vi "ApplicaFunzCorr_INPUT.vi"(0 "Array":T1[](array[typedef])) -> (7 "Array Cluster Corretto":T1[](array[typedef]))   [LabVIEW 2016]
uses:
  <vilib>/Analysis/6fits.llb/Curve Fitting Criteria.ctl
  <vilib>/Utility/file.llb/Read Delimited Spreadsheet (string).vi
  <vilib>/Analysis/polynomials.llb/Scalar Polynomial Evaluation (DBL).vi
  <vilib>/Analysis/polynomials.llb/Polynomial Plot (Range).vi
  <vilib>/Analysis/NI_AALPro.lvlib
panel:
  in  "Cluster Misura / Unità":T1
  out "Misure da correggere":dbl[](array[numeric])
  out "Misure Corrette":dbl[](array[numeric])
  out "Graph":cluster{"Ramp Pattern":dbl[], "P(A)":dbl[]}[](graph)
  out "Y":dbl[](array[numeric])
  out "X":dbl[](array[numeric])
  out "Subarray dati selezionati":string[][](array[string])
  out "Lettura file di testo":string[][](array[string])
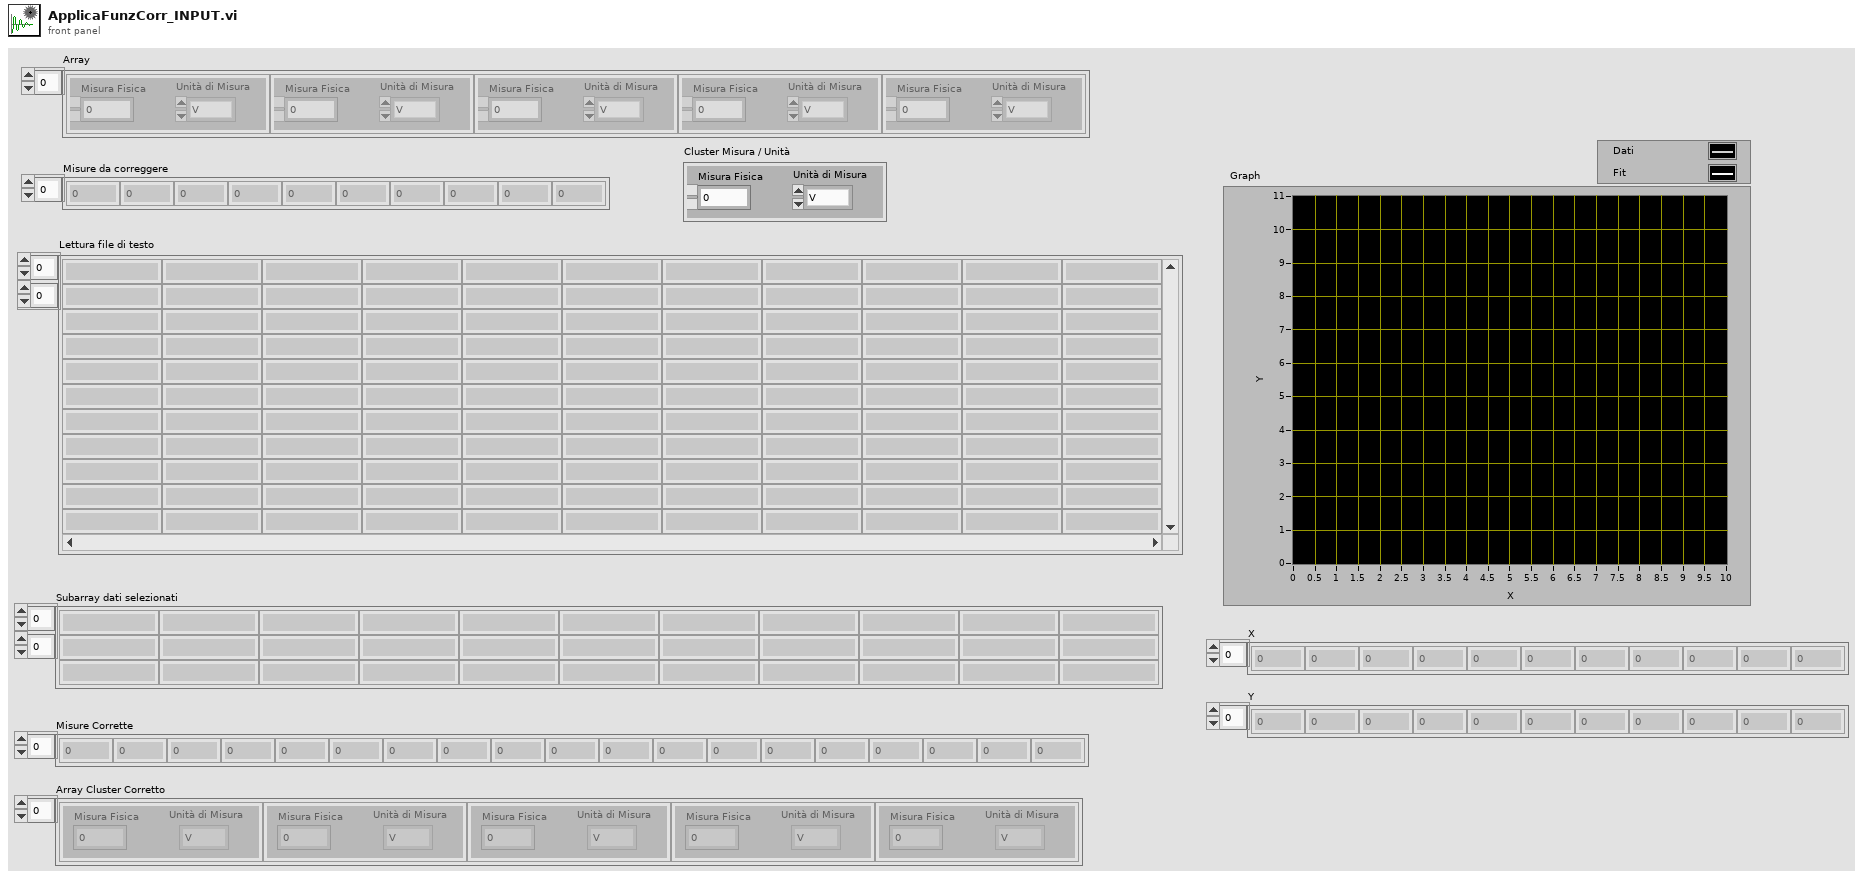
[diagram p1: front panel]
types:
  T1 = typedef "ClusterMisura_e_Unità_INPUT.ctl" = cluster{"Misura Fisica":dbl, "Unità di Misura":T2}
  T2 = typedef "UnitàMisura.ctl" = enum16{"V", "mA", "Bar", "RPM", "m3/s", "m3/min", "m3/h", "l/s", "l/min", "in3/min", "ft3/min", "gpm", "igpm", "igph"}
  T3 = typedef "NI_AALPro.lvlib/Curve Fitting Criteria.ctl" = u16
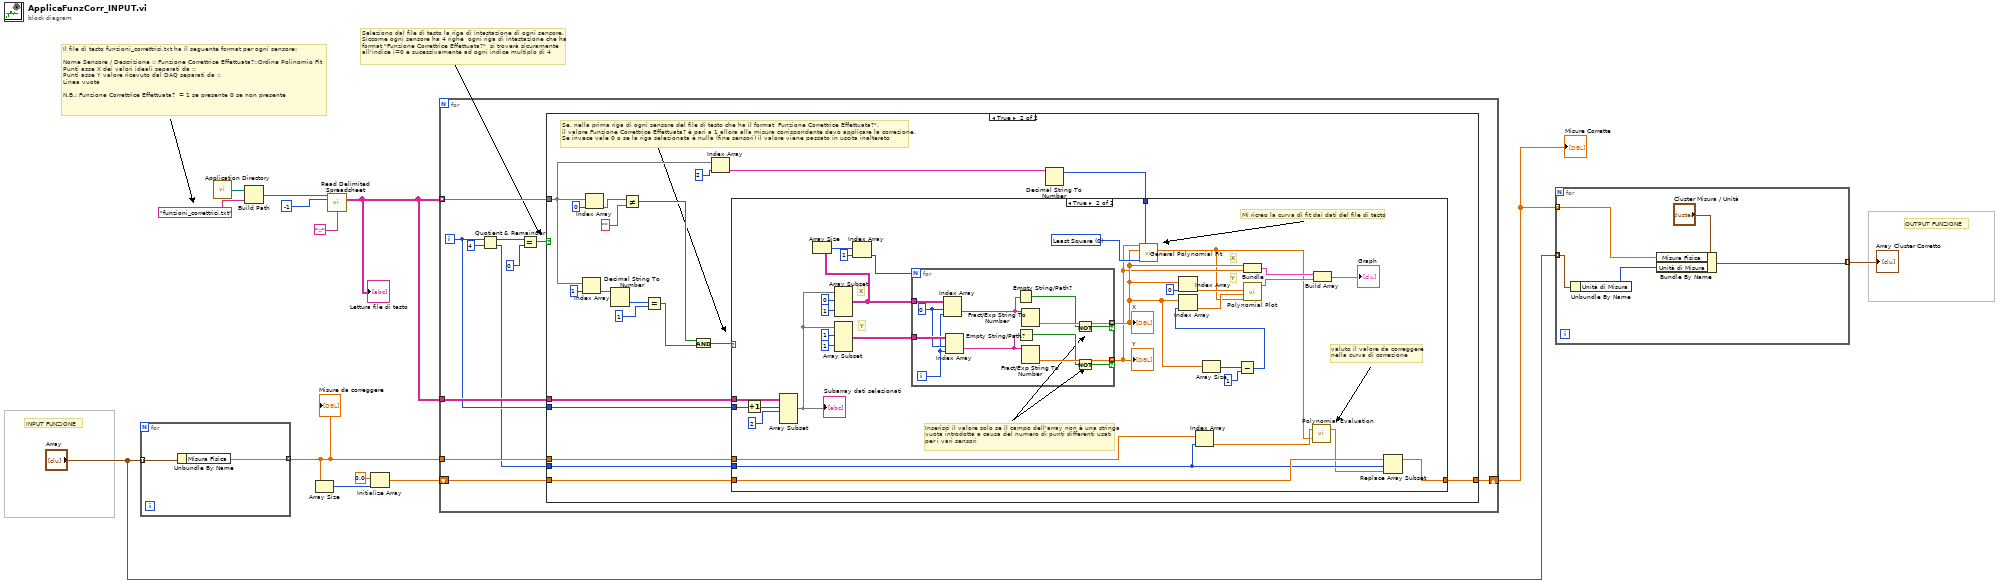
[diagram p0: block diagram]
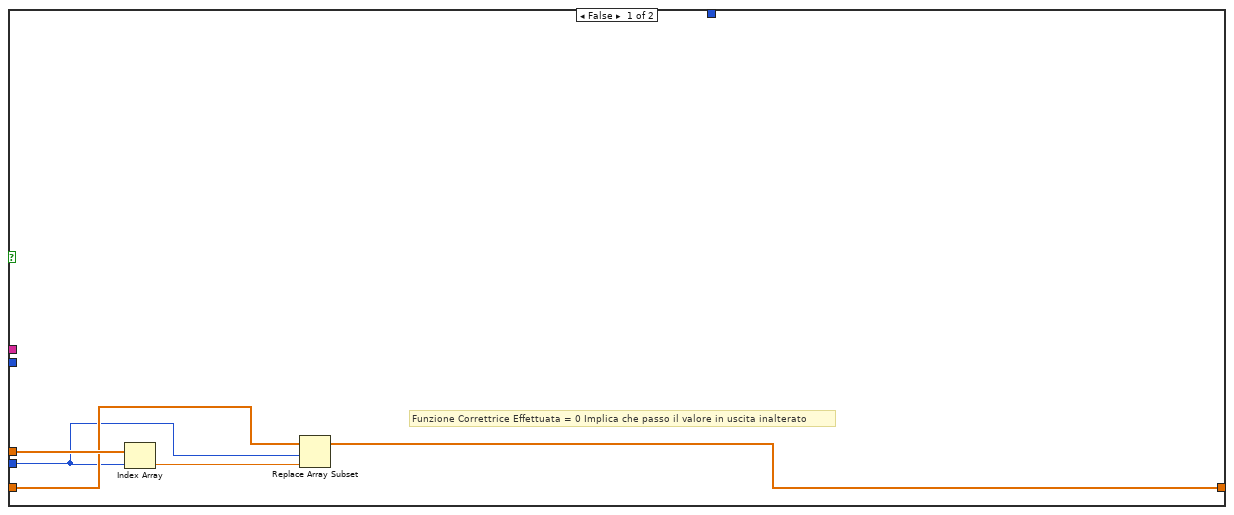
[diagram p3: hidden frame]
diagram:
  # "Seleziono dal file di testo la riga di intestazione di ogni sensore. \nSiccome ogni sensore ha 4 righe  ogni riga di intestazione che ha \nformat \"Funzione Correttrice Effettuata?\"  si troverà sicuramente \nall'indice i=0 e sucessivamente ad ogni indice multiplo di 4"
  # "Il file di testo funzioni_correttrici.txt ha il seguente format per ogni sensore:\n\nNome Sensore / Descrizione :: Funzione Correttrice Effettuata?::Ordine Polinomio Fit \nPunti asse X dei valori ideali separati da ::\nPunti asse Y valore ricevuto dal DAQ separati da ::\nLinea vuota\n\nN.B.: Funzione Correttrice Effettuata?  = 1 se presente 0 se non presente"
  # "OUTPUT FUNZIONE"
  # "INPUT FUNZIONE"
  n1 = for {
    tunnel: "Array" -> [w15] mode=indexing
    tunnel: [w14] -> w4 mode=indexing
    n2 = Unbundle By Name(w15) -> ("Misura Fisica"=w14:dbl)
  }
  "Misure da correggere" <- w4
  n3 = call <vilib>:"Application Directory.vi"() -> ("Application Directory"=w12:path)
  n4 = Build Path(base path=w12, name or relative path="funzioni_correttrici.txt") -> (appended path=w11:path)
  n5 = Array Size(array=w4) -> (size(s)=w7:i32)
  n6 = call-poly <vilib>:"Read Delimited Spreadsheet.vi"("file path (dialog if empty)"=w11, "number of rows (all:-1)"=-1, "delimiter (\\t)"="::" ("delimiter (\\t)")) -> ("all rows"=w8:string[][])  [unwired: 7 in, 5 out]
  "Lettura file di testo" <- w8
  n7 = Initialize Array(0.0 ("element"), w7) -> (w5:dbl[])
  n8 = for {
    tunnel: w8 -> [w22] mode=indexing
    tunnel: w8 -> [w21]
    tunnel: w4 -> [w19]
    shift-right: [w17] -> w2
    shift-left: w5 -> [w16]
    i -> [w20]
    n9 = Quotient & Remainder(x=w20, y=4) -> (x-y*floor(x/y)=w25:i32, floor(x/y)=w18:i32)
    n10 = Equal?(x=w25, y=0) -> (x = y?=w23:bool)
    n11 = case shown="True" w23 {
      tunnel: w22 -> [_ w31]
      tunnel: w21 -> [_ w37]
      tunnel: w20 -> [_ w36]
      tunnel: w19 -> [_ w35]
      tunnel: w18 -> [_ w34]
      tunnel: w16 -> [w27 w33]
      tunnel: [w27 w32] -> w17
      frame False {
      }
      frame True {
        # "Se, nella prima riga di ogni sensore del file di testo che ha il format  Funzione Correttrice Effettuata?\",\nil valore Funzione Correttrice Effettuata? è pari a 1 allora alla misura corrispondente devo applicare la correzione.\nSe invece vale 0 o se la riga selezionata è nulla (fine sensori) il valore viene passato in uscita inalterato"
        n12 = Index Array(array=w31, index=1) -> (element=w46:string)
        n13 = Index Array(array=w31, index=0) -> (element=w40:string)
        n14 = Decimal String To Number(string=w46) -> (number=w45:i32)  [unwired: 2 in, 1 out]
        n15 = Not Equal?(x=w40, y="") -> (x != y?=w41:bool)
        n16 = Equal?(x=w45, y=1) -> (x = y?=w42:bool)
        n17 = And(x=w41, y=w42) -> (x .and. y?=w43:bool)
        n18 = Index Array(array=w31, index=2) -> (element=w29:string)
        n19 = Decimal String To Number(string=w29) -> (offset past number=w28:i32)  [unwired: 2 in, 1 out]
        n20 = case shown="True" w43 {
          tunnel: w37 -> [_ w84]
          tunnel: w36 -> [_ w85]
          tunnel: w35 -> [w52 w60]
          tunnel: w34 -> [w49 w56]
          tunnel: w33 -> [w51 w57]
          tunnel: [w48 w58] -> w32
          tunnel: w28 -> [_ w53]
          frame False {
            # "Funzione Correttrice Effettuata = 0 Implica che passo il valore in uscita inalterato"
            n21 = Index Array(array=w52, index=w49) -> (element=w50:dbl)
            n22 = Replace Array Subset(array=w51, new element=w50, index=w49) -> (w48:dbl[])
          }
          frame True {
            w86 = T3 0 items=["Least Square", "Least Absolute Residual", "Bisquare"] ("method")
            # "valuto il valore da correggere\nnella curva di correzione"
            # "Mi ricreo la curva di fit dai dati del file di testo"
            # "Y"
            # "X"
            # "Inserisci il valore solo se il campo dell'array non è una stringa\nvuota introdotta a causa del numero di punti differenti usati \nper i vari sensori"
            # "Y"
            # "X"
            n23 = Increment(x=w85) -> (x+1=w83:i32)
            n24 = Array Subset(array=w84, index (row)=w83, length (row)=2 ("length")) -> (w79:string[][])  [unwired: 2 in]
            "Subarray dati selezionati" <- w79
            n25 = Array Subset(array=w79, index (row)=0 ("index"), length (row)=1 ("length")) -> (w75:string[][])  [unwired: 2 in]
            n26 = Array Size(array=w75) -> (size(s)=w74:i32[])
            n27 = Array Subset(array=w79, index (row)=1 ("index"), length (row)=1 ("length")) -> (w76:string[][])  [unwired: 2 in]
            n28 = Index Array(array=w74, index=1) -> (element=w72:i32)
            n29 = for {
              N: w72 -> [_]
              tunnel: w75 -> [w96]
              tunnel: w76 -> [w95]
              tunnel: [w98] -> w65 mode=indexing if=w90
              tunnel: [w97] -> w64 mode=indexing if=w89
              i -> [w93]
              w94 = 0 ("index (row)")
              n30 = Index Array(array=w96, index (row)=w94, index (col)=w93) -> (element=w92:string)
              n31 = Index Array(array=w95, index (row)=w94, index (col)=w93) -> (element=w87:string)
              n32 = Empty String/Path?(string/path=w92) -> (empty?=w91:bool)
              n33 = Empty String/Path?(string/path=w87) -> (empty?=w88:bool)
              n34 = Fract/Exp String To Number(string=w92) -> (number=w98:dbl)  [unwired: 3 in, 1 out]
              n35 = Fract/Exp String To Number(string=w87) -> (number=w97:dbl)  [unwired: 3 in, 1 out]
              n36 = Not(x=w91) -> (.not. x?=w90:bool)
              n37 = Not(x=w88) -> (.not. x?=w89:bool)
            }
            "X" <- w65
            "Y" <- w64
            n38 = call <vilib>:"General Polynomial Fit.vi"("Y"=w64, "polynomial order"=w53, "X"=w65, "method"=w86) -> ("Polynomial Coefficients"=w54:dbl[])  [unwired: 8 in, 3 out]
            n39 = Index Array(array=w65, index=0) -> (element=w66:dbl)
            n40 = Index Array(array=w60, index=w56) -> (element=w59:dbl)
            n41 = Array Size(array=w65) -> (size(s)=w70:i32)
            n42 = Subtract(x=w70, y=1) -> (x-y=w68:i32)
            n43 = Index Array(array=w65, index=w68) -> (element=w67:dbl)
            n44 = call-poly <vilib>:"Polynomial Plot.vi"("P(x)"=w54, "end"=w67, "start"=w66) -> ("polynomial plot"=w62:cluster{"Ramp Pattern":dbl[], "P(A)":dbl[]})  [unwired: 7 in, 1 out]
            n45 = Bundle(w65, w64) -> (w63:cluster{dbl[], dbl[]})  [unwired: 1 in]
            n46 = call-poly <vilib>:"Polynomial Evaluation.vi"("P(x)"=w54, "a"=w59) -> ("P(a)"=w55:dbl)  [unwired: 1 out]
            n47 = Build Array(w63, w62) -> (→"Graph":cluster{"Ramp Pattern":dbl[], "P(A)":dbl[]}[])
            n48 = Replace Array Subset(array=w57, new element=w55, index=w56) -> (w58:dbl[])
          }
        }
      }
    }
  }
  "Misure Corrette" <- w2
  n49 = for {
    tunnel: "Array" -> [w101] mode=indexing
    tunnel: w2 -> [w102] mode=indexing
    tunnel: [w99] -> w1 mode=indexing
    n50 = Unbundle By Name(w101) -> ("Unità di Misura"=w100:T2)
    n51 = Bundle By Name(cluster="Cluster Misura / Unità", "Misura Fisica"=w102, "Unità di Misura"=w100) -> (w99:T1)
  }
  "Array Cluster Corretto" <- w1
